vi "Main.vi"(11 "Module Admin":refnum<class "Delacor_lib_QMH_Module Admin.lvclass">) -> ()   [LabVIEW 2020, in "Manipulator.lvlib"]
doc: "This template is based off of the Queued Message Handler design pattern and the Queued Message Handler project template that ships with LabVIEW.\n\nThe main difference is that the queue is private to this module and communication between modules is performed via Broadcast and Request events.\n\nRequest events are wrapped in public API methods and are handled in the Event Handling Loop (EHL) of this VI. Any module can register for Broadcast events sent by this module. The EHL generates messages based on user interface actions.\n\nThe Message Handling Loop (MHL) processes messages generated by the EHL, or by other messages. The messages are string values, so new messages can be added easily to the Message Cases case structure in the MHL. Each message cluster can also provide an optional value for Message Data, which is a variant that can be converted to whatever message-specific data is required.\n_____\nBased on DQMH Project Template 6.0.0.91."
uses:
  Manipulator.lvlib
  <vilib>/Delacor/Delacor QMH/Libraries/Module Admin_class/Delacor_lib_QMH_Module Admin.lvclass
  Module Data--cluster.ctl
  <vilib>/Delacor/Delacor QMH/Libraries/Message Queue_class/Delacor_lib_QMH_Message Queue.lvclass/Delacor_lib_QMH_Message Queue.ctl
  Stop Argument--cluster.ctl
  <vilib>/Delacor/Delacor QMH/Libraries/Module Admin_class/Delacor_lib_QMH_Module Admin.lvclass/Delacor_lib_QMH_Module Admin.ctl
  Get Num Axes Argument--cluster.ctl
  Get Num Axes (Reply Payload)--cluster.ctl
  Get Position and Speed Argument--cluster.ctl
  Get Position and Speed (Reply Payload)--cluster.ctl
  Move Axis Argument--cluster.ctl
  Move Axis (Reply Payload)--cluster.ctl
  Get Status Argument--cluster.ctl
  Get Status (Reply Payload)--cluster.ctl
  Manipulator-CLIDriver/Manipulator Status.ctl
  Move Axis with Speed Argument--cluster.ctl
  Move Axis with Speed (Reply Payload)--cluster.ctl
  <vilib>/Utility/miscctls.llb/LVPointTypeDef.ctl
  <vilib>/Delacor/Delacor QMH/Libraries/Message Queue_class/Delacor_lib_QMH_Enqueue Message (Single).vi
  <vilib>/Delacor/Delacor QMH/Libraries/Module Admin_class/Delacor_lib_QMH_Get External Launch.vi
  <vilib>/Utility/error.llb/Error Cluster From Error Code.vi
  <vilib>/ErrorRing/Error Ring.xnode
  <vilib>/Delacor/Delacor QMH/Libraries/Message Queue_class/Delacor_lib_QMH_Message Queue.lvclass
  Manipulator-CLIDriver/Manipulator CLI Driver.lvlib
panel:
  out "error out":errorcluster
  out "Status":string
  in  "Simulate MHL Error":bool
  in  "Simulate EHL Error":bool
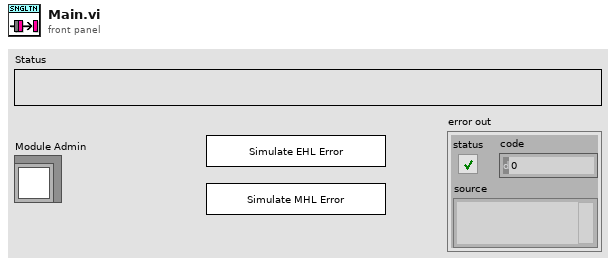
[diagram p1: front panel]
types:
  T1 = typedef "Manipulator.lvlib/Request Events--cluster.ctl" = cluster{"Stop Module":refnum<user-event>, "Show Panel":refnum<user-event>, "Hide Panel":refnum<user-event>, "Get Module Execution Status":refnum<user-event>, "Show Diagram":refnum<user-event>, "Get Num Axes":refnum<user-event>, "Get Position and Speed":refnum<user-event>, "Move Axis":refnum<user-event>, "Get Status":refnum<user-event>, "Move Axis with Speed":refnum<user-event>}
  T2 = typedef "Manipulator.lvlib/Module Data--cluster.ctl" = cluster{"Status":string}
  T3 = enum32{"invalid lock state", "Not Locked", "Locked (No Password)", "Password-protected"}
  T4 = typedef "Manipulator.lvlib/Stop Argument--cluster.ctl" = cluster{"Origin":string, "Exit via Stop Module Req?":bool, "Wait for Module to stop?":bool}
  T5 = typedef "Manipulator.lvlib/Get Num Axes Argument--cluster.ctl" = cluster{"Wait Notifier":refnum<notifier>, "wait for reply":bool}
  T6 = typedef "Manipulator.lvlib/Get Position and Speed Argument--cluster.ctl" = cluster{"Wait Notifier":refnum<notifier>, "wait for reply":bool}
  T7 = typedef "Manipulator.lvlib/Move Axis Argument--cluster.ctl" = cluster{"Axis":i32, "Position":dbl, "Wait Notifier":refnum<notifier>, "wait for reply":bool}
  T8 = typedef "Manipulator.lvlib/Get Status Argument--cluster.ctl" = cluster{"Wait Notifier":refnum<notifier>, "wait for reply":bool}
  T9 = typedef "Manipulator.lvlib/Move Axis with Speed Argument--cluster.ctl" = cluster{"Position":dbl, "Speed":dbl, "Axis":i32, "Wait Notifier":refnum<notifier>, "wait for reply":bool}
  T10 = typedef "LVPointTypeDef.ctl" = cluster{"Horizontal":i16, "Vertical":i16}
  T11 = enum32{"Invalid", "Standard", "Closed", "Hidden", "Minimized", "Maximized"}
  T12 = typedef "Manipulator.lvlib/Get Num Axes (Reply Payload)--cluster.ctl" = cluster{"Num Axes":i32, "Get Num Axes_error":errorcluster}
  T13 = typedef "Manipulator.lvlib/Get Position and Speed (Reply Payload)--cluster.ctl" = cluster{"Positions":dbl[], "Speeds":dbl[], "Get Position and Speed_error":errorcluster}
  T14 = typedef "Manipulator.lvlib/Move Axis (Reply Payload)--cluster.ctl" = cluster{"Move Axis_error":errorcluster}
  T15 = typedef "Manipulator.lvlib/Get Status (Reply Payload)--cluster.ctl" = cluster{"Status":T16, "Get Status_error":errorcluster}
  T16 = typedef "Manipulator CLI Driver.lvlib/Manipulator Status.ctl" = enum16{"Moving", "Done", "Aborted", "Error", "No Status"}
  T17 = typedef "Manipulator.lvlib/Move Axis with Speed (Reply Payload)--cluster.ctl" = cluster{"Move Axis with Speed_error":errorcluster}
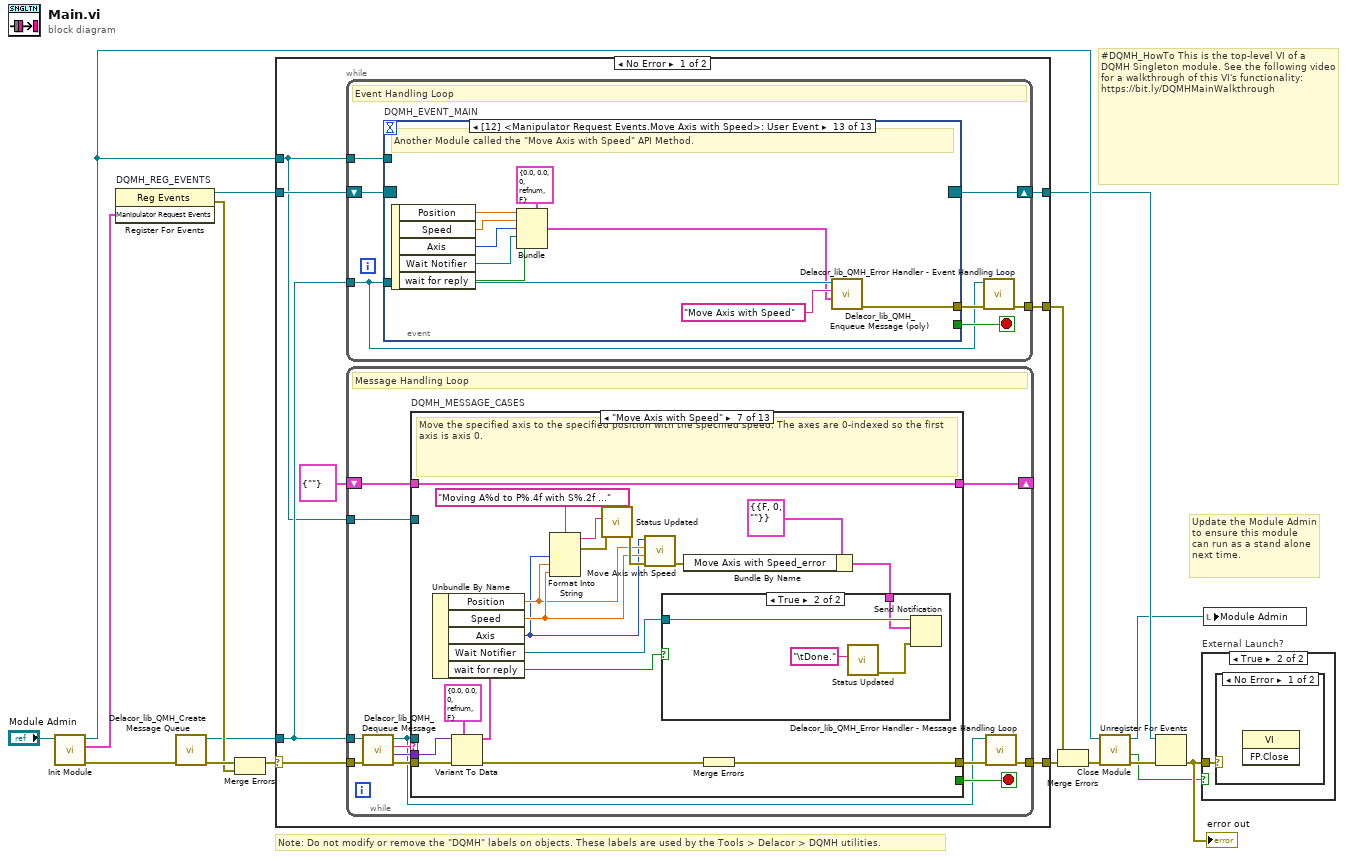
[diagram p0: block diagram]
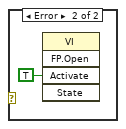
[diagram p3: hidden frame]
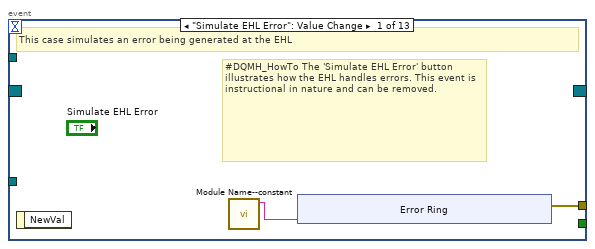
[diagram p4: hidden frame]
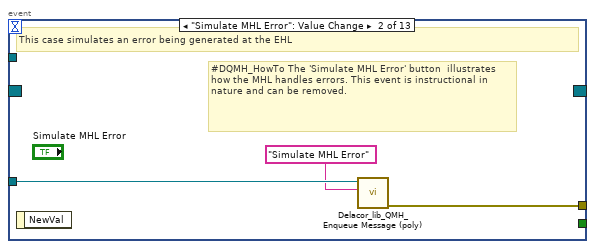
[diagram p5: hidden frame]
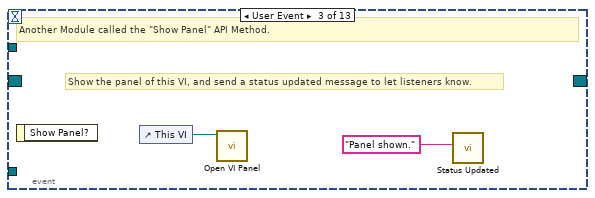
[diagram p6: hidden frame]
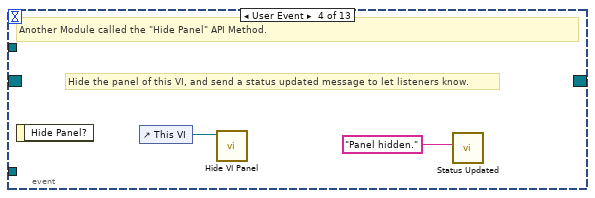
[diagram p7: hidden frame]
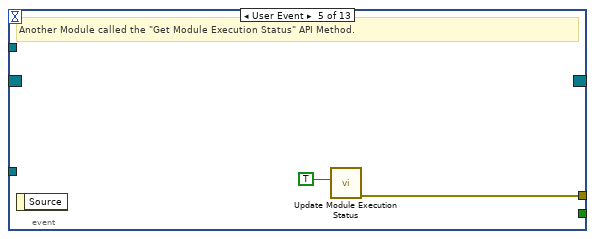
[diagram p8: hidden frame]
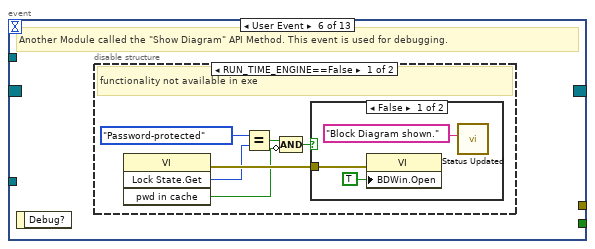
[diagram p9: hidden frame]
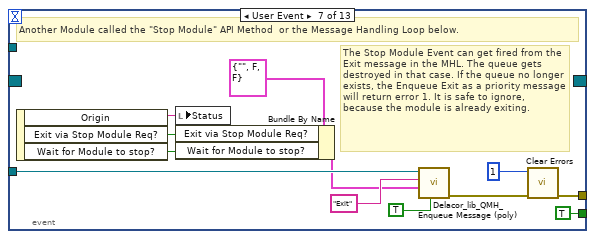
[diagram p12: hidden frame]
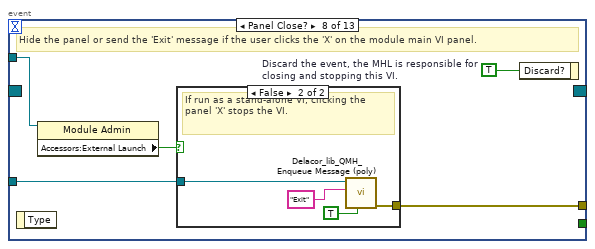
[diagram p13: hidden frame]
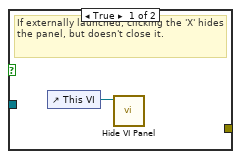
[diagram p14: hidden frame]
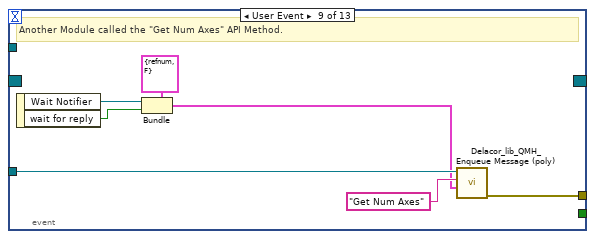
[diagram p15: hidden frame]
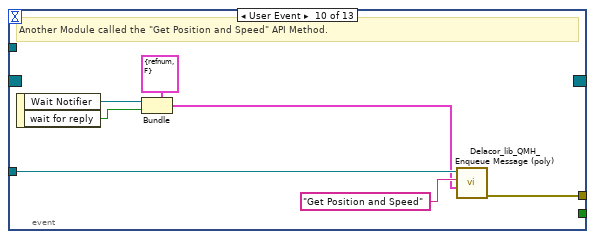
[diagram p16: hidden frame]
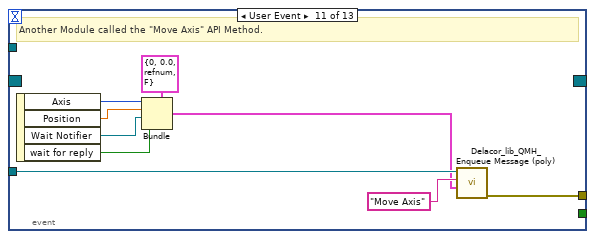
[diagram p17: hidden frame]
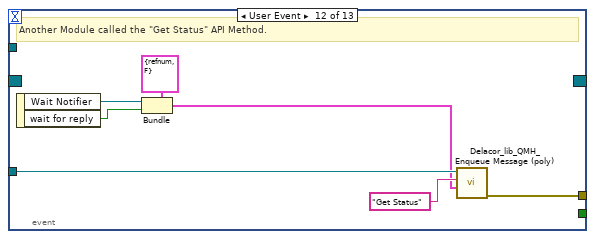
[diagram p18: hidden frame]
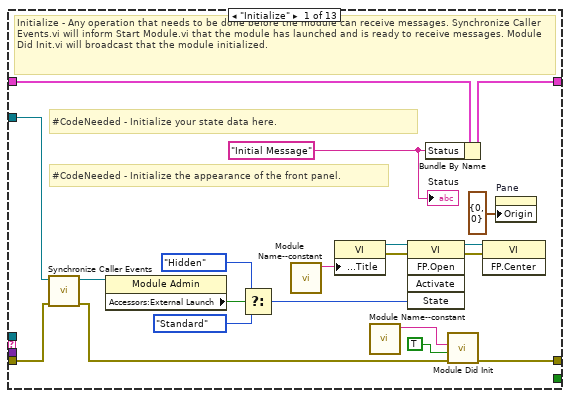
[diagram p19: hidden frame]
diagram:
  # "#DQMH_HowTo This is the top-level VI of a DQMH Singleton module. See the following video for a walkthrough of this VI's functionality: https://bit.ly/DQMHMainWalkthrough"
  # "Note: Do not modify or remove the \"DQMH\" labels on objects. These labels are used by the Tools > Delacor > DQMH utilities."
  # "Update the Module Admin to ensure this module can run as a stand alone next time."
  n1 = call "Init Module.vi"("Singleton Module Admin in"="Module Admin") -> ("error out"=w16:errorcluster, "Manipulator Request Events"=w5:T1, "Singleton Module Admin out"=w8:refnum<class "Delacor_lib_QMH_Module Admin.lvclass">)  [unwired: 8 in]
  n2 = register-events "DQMH_REG_EVENTS"(w5) -> (reference out=w6:refnum<event-registration>, error out=w9:errorcluster)  [unwired: 2 in]
  n3 = call <vilib>:"Delacor_lib_QMH_Create Message Queue.vi"("error in"=w16) -> ("error out"=w11:errorcluster, "Message Queue"=w4:refnum<class "Delacor_lib_QMH_Message Queue.lvclass">)  [unwired: 9 in]
  n4 = Merge Errors(w11, w9) -> (w10:errorcluster)
  n5 = case shown="No Error" w10 {
    selector: w10 -> [w23 w311]
    tunnel: [w25 w310] -> w17
    tunnel: [w22 w316] -> w7
    tunnel: w6 -> [w20 w316]
    tunnel: w4 -> [w19 w309]
    tunnel: [w24 _] -> w14
    tunnel: w8 -> [w18 w312]
    frame No Error {
      n6 = while {
        tunnel: w19 -> [w26]
        shift-right: [w29] -> w22
        shift-left: w20 -> [w30]
        tunnel: [w31] -> w24
        tunnel: w18 -> [w27]
        stop <- w28 stop-if-true
        # "Event Handling Loop"
        n7 = event "DQMH_EVENT_MAIN" shown="[12] <Manipulator Request Events.Move Axis with Speed>: User Event" {
          selector: w30 -> [_ _ _ _ _ _ _ _ _ _ _ _ _]
          dyn-events: [_ _ _ _ _ _ _ _ _ _ _ _ _] -> w29
          timeout: _ -> [_ _ _ _ _ _ _ _ _ _ _ _ _]
          tunnel: [_ _ _ _ _ _ TRUE ("Discard?") _ _ _ _ _ _] -> w28
          tunnel: w26 -> [_ w43 _ _ _ _ w67 w74 w88 w95 w104 w111 w121]
          tunnel: [w34 w44 _ _ w50 _ w70 w76 w82 w89 w96 w105 w112] -> w32
          tunnel: w27 -> [_ _ _ _ _ _ _ w73 _ _ _ _ _]
          event "Simulate EHL Error": Value Change {
            # "#DQMH_HowTo The 'Simulate EHL Error' button  illustrates how the EHL handles errors. This event is instructional in nature and can be removed."
            # "This case simulates an error being generated at the EHL"
            n8 = event-data() -> ()  [unwired: 1 in, 1 out]
            n9 = call "Module Name--constant.vi"() -> ("Module Name"=w33:string)  [unwired: 11 in]
            n10 = xnode "Error Ring"("parameter 0"=w33) -> ("error out"=w34:errorcluster)
          }
          event "Simulate MHL Error": Value Change {
            # "#DQMH_HowTo The 'Simulate MHL Error' button  illustrates how the MHL handles errors. This event is instructional in nature and can be removed."
            # "This case simulates an error being generated at the EHL"
            n11 = event-data() -> ()  [unwired: 1 in, 1 out]
            n12 = call-poly <vilib>:"Delacor_lib_QMH_Enqueue Message (poly).vi"("Message"="Simulate MHL Error", "Message Queue in"=w43) -> ("error out"=w44:errorcluster)  [unwired: 8 in, 1 out]
          }
          event User Event {
            # "Show the panel of this VI, and send a status updated message to let listeners know."
            # "Another Module called the \"Show Panel\" API Method."
            n13 = event-data() -> ()  [unwired: 1 in, 1 out]
            n14 = control-ref of="This VI"() -> (w46:refnum<vi>)
            n15 = call "Open VI Panel.vi"("VI"=w46) -> ()  [unwired: 10 in, 1 out]
            n16 = call "Status Updated.vi"("Status"="Panel shown." ("format string")) -> ()  [unwired: 10 in, 1 out]
          }
          event User Event {
            # "Hide the panel of this VI, and send a status updated message to let listeners know."
            # "Another Module called the \"Hide Panel\" API Method."
            n17 = event-data() -> ()  [unwired: 1 in, 1 out]
            n18 = control-ref of="This VI"() -> (w48:refnum<vi>)
            n19 = call "Hide VI Panel.vi"("VI"=w48) -> ()  [unwired: 10 in, 1 out]
            n20 = call "Status Updated.vi"("Status"="Panel hidden." ("format string")) -> ()  [unwired: 10 in, 1 out]
          }
          event User Event {
            # "Another Module called the \"Get Module Execution Status\" API Method."
            n21 = event-data() -> ()  [unwired: 1 in, 1 out]
            n22 = call "Update Module Execution Status.vi"("Running?"=TRUE) -> ("error out"=w50:errorcluster)  [unwired: 10 in]
          }
          event User Event {
            # "Another Module called the \"Show Diagram\" API Method. This event is used for debugging."
            n23 = event-data() -> ()  [unwired: 1 in, 1 out]
            n24 = disable-structure shown="RUN_TIME_ENGINE==False" {
              frame condition #0 (active) {
                # "functionality not available in exe"
                n25 = invoke class="VI" method="Lock State.Get"() -> (error out=w56:errorcluster, "Get Lock State"=w55:T3, "pwd in cache"=w52:bool)  [unwired: 4 in, 1 out]
                n26 = Equal?(x=T3."Password-protected", y=w55) -> (x = y?=w53:bool)
                n27 = Compound Arithmetic op=AND(w53, invert w52) -> (w51:bool)
                n28 = case shown="False" w51 {
                  tunnel: w56 -> [w59 _]
                  frame False {
                    n29 = property class="VI"(error in=w59, "BDWin.Open"=TRUE ("Block Diagram Window:Open")) -> ()  [unwired: 1 in, 2 out]
                    n30 = call "Status Updated.vi"("Status"="Block Diagram shown." ("format string")) -> ()  [unwired: 10 in, 1 out]
                  }
                  frame True {
                    # "Password-protected VI, and the password is not in the cache. Do not show the diagram."
                  }
                }
              }
              frame condition #1 {
              }
            }
          }
          event User Event {
            # "The Stop Module Event can get fired from the Exit message in the MHL. The queue gets destroyed in that case. If the queue no longer exists, the Enqueue Exit as a priority message will return error 1. It is safe to ignore, because the module is already exiting."
            # "Another Module called the \"Stop Module\" API Method  or the Message Handling Loop below."
            n31 = event-data() -> ("Origin"=w66:string, "Exit via Stop Module Req?"=w62:bool, "Wait for Module to stop?"=w61:bool)  [unwired: 1 in]
            n32 = local write "Status"(w66) -> ()
            n33 = Bundle By Name(cluster=T4 {"Origin"="", "Exit via Stop Module Req?"=FALSE, "Wait for Module to stop?"=FALSE} ("Stop Argument"), "Exit via Stop Module Req?"=w62, "Wait for Module to stop?"=w61) -> (w60:T4)
            n34 = call-poly <vilib>:"Delacor_lib_QMH_Enqueue Message (poly).vi"("Priority Message? (F)"=TRUE, "Message Data"=w60, "Message"="Exit", "Message Queue in"=w67) -> ("error out"=w71:errorcluster)  [unwired: 6 in, 1 out]
            n35 = call <vilib>:"Clear Errors.vi"("error in (no error)"=w71, "specific error code to clear (0: all)"=1) -> ("error out"=w70:errorcluster)  [unwired: 4 in, 1 out]
          }
          event Panel Close? {
            w75 = TRUE  # Discard the event, the MHL is responsible for closing and stopping this VI.
            # "Hide the panel or send the 'Exit' message if the user clicks the 'X' on the module main VI panel."
            n36 = event-data() -> ()  [unwired: 1 in, 1 out]
            n37 = property class="Module Admin"(reference=w73) -> ("Accessors:External Launch"=w72:bool)  [unwired: 1 in, 2 out]
            n38 = case shown="False" w72 {
              tunnel: w74 -> [_ w80]
              tunnel: [_ w81] -> w76
              frame True {
                # "If externally launched, clicking the 'X' hides the panel, but doesn't close it."
                n39 = control-ref of="This VI"() -> (w77:refnum<vi>)
                n40 = call "Hide VI Panel.vi"("VI"=w77) -> ()  [unwired: 10 in, 1 out]
              }
              frame False {
                # "If run as a stand-alone VI, clicking the panel 'X' stops the VI."
                n41 = call-poly <vilib>:"Delacor_lib_QMH_Enqueue Message (poly).vi"("Priority Message? (F)"=TRUE, "Message"="Exit", "Message Queue in"=w80) -> ("error out"=w81:errorcluster)  [unwired: 7 in, 1 out]
              }
            }
            n42 = event-data("Discard?"=w75) -> ()  [unwired: 1 in, 1 out]
          }
          event User Event {
            # "Another Module called the \"Get Num Axes\" API Method."
            n43 = event-data() -> ("Wait Notifier"=w84:refnum<notifier>, "wait for reply"=w83:bool)  [unwired: 1 in]
            n44 = Bundle(cluster=T5 {"Wait Notifier"=refnum, "wait for reply"=FALSE} ("Get Num Axes Argument"), "Wait Notifier"=w84, "wait for reply"=w83) -> (w85:T5)
            n45 = call-poly <vilib>:"Delacor_lib_QMH_Enqueue Message (poly).vi"("Message Data"=w85, "Message"="Get Num Axes", "Message Queue in"=w88) -> ("error out"=w82:errorcluster)  [unwired: 7 in, 1 out]
          }
          event User Event {
            # "Another Module called the \"Get Position and Speed\" API Method."
            n46 = event-data() -> ("Wait Notifier"=w91:refnum<notifier>, "wait for reply"=w90:bool)  [unwired: 1 in]
            n47 = Bundle(cluster=T6 {"Wait Notifier"=refnum, "wait for reply"=FALSE} ("Get Position and Speed Argument"), "Wait Notifier"=w91, "wait for reply"=w90) -> (w92:T6)
            n48 = call-poly <vilib>:"Delacor_lib_QMH_Enqueue Message (poly).vi"("Message Data"=w92, "Message"="Get Position and Speed", "Message Queue in"=w95) -> ("error out"=w89:errorcluster)  [unwired: 7 in, 1 out]
          }
          event User Event {
            # "Another Module called the \"Move Axis\" API Method."
            n49 = event-data() -> ("Axis"=w100:i32, "Position"=w99:dbl, "Wait Notifier"=w98:refnum<notifier>, "wait for reply"=w97:bool)  [unwired: 1 in]
            n50 = Bundle(cluster=T7 {"Axis"=0, "Position"=0.0, "Wait Notifier"=refnum, "wait for reply"=FALSE} ("Move Axis Argument"), "Axis"=w100, "Position"=w99, "Wait Notifier"=w98, "wait for reply"=w97) -> (w101:T7)
            n51 = call-poly <vilib>:"Delacor_lib_QMH_Enqueue Message (poly).vi"("Message Data"=w101, "Message"="Move Axis", "Message Queue in"=w104) -> ("error out"=w96:errorcluster)  [unwired: 7 in, 1 out]
          }
          event User Event {
            # "Another Module called the \"Get Status\" API Method."
            n52 = event-data() -> ("Wait Notifier"=w107:refnum<notifier>, "wait for reply"=w106:bool)  [unwired: 1 in]
            n53 = Bundle(cluster=T8 {"Wait Notifier"=refnum, "wait for reply"=FALSE} ("Get Status Argument"), "Wait Notifier"=w107, "wait for reply"=w106) -> (w108:T8)
            n54 = call-poly <vilib>:"Delacor_lib_QMH_Enqueue Message (poly).vi"("Message Data"=w108, "Message"="Get Status", "Message Queue in"=w111) -> ("error out"=w105:errorcluster)  [unwired: 7 in, 1 out]
          }
          event User Event {
            # "Another Module called the \"Move Axis with Speed\" API Method."
            n55 = event-data() -> ("Position"=w117:dbl, "Speed"=w116:dbl, "Axis"=w115:i32, "Wait Notifier"=w114:refnum<notifier>, "wait for reply"=w113:bool)  [unwired: 1 in]
            n56 = Bundle(cluster=T9 {"Position"=0.0, "Speed"=0.0, "Axis"=0, "Wait Notifier"=refnum, "wait for reply"=FALSE} ("Move Axis with Speed Argument"), "Position"=w117, "Speed"=w116, "Axis"=w115, "Wait Notifier"=w114, "wait for reply"=w113) -> (w118:T9)
            n57 = call-poly <vilib>:"Delacor_lib_QMH_Enqueue Message (poly).vi"("Message Data"=w118, "Message"="Move Axis with Speed", "Message Queue in"=w121) -> ("error out"=w112:errorcluster)  [unwired: 7 in, 1 out]
          }
        }
        n58 = call-dynamic "Delacor_lib_QMH_Error Handler - Event Handling Loop.vi"("error in"=w32, "Message Queue in"=w26) -> ("dup error in"=w31:errorcluster)  [unwired: 8 in, 1 out]
      }
      n59 = while {
        tunnel: w19 -> [w124]
        shift-right: [w128] -> _
        shift-left: T2 {"Status"=""} ("Data Cluster") -> [w129]
        tunnel: w23 -> [w132]
        tunnel: [w130] -> w25
        tunnel: w18 -> [w122]
        stop <- w127 stop-if-true
        # "Message Handling Loop"
        n60 = call-dynamic "Delacor_lib_QMH_Dequeue Message.vi"("error in"=w132, "Message Queue in"=w124) -> ("error out"=w131:errorcluster, "Message Data"=w125:variant, "Message"=w126:string, "Message Queue out"=w123:refnum<class "Delacor_lib_QMH_Message Queue.lvclass">)  [unwired: 6 in]
        n61 = case "DQMH_MESSAGE_CASES" shown="\"Move Axis with Speed\"" w126 {
          selector: w126 -> [_ _ _ _ _ _ _ _ _ _ _ _ w296]
          tunnel: w123 -> [_ _ _ _ _ _ _ _ _ _ w266 w288 _]
          tunnel: w131 -> [w151 w155 w168 w184 w204 w221 w242 w249 w251 w256 w273 w294 w298]
          tunnel: [w149 w155 w158 w174 w194 w211 w232 w248 w251 w255 w269 w291 w299] -> w133
          tunnel: w129 -> [w140 w154 w167 w183 w203 w220 w241 w247 w250 w253 w268 w287 w297]
          tunnel: [w139 w154 w167 w183 w203 w220 w241 w247 w250 w253 w268 w287 w297] -> w128
          tunnel: [_ _ _ _ _ _ _ _ _ _ _ w286 _] -> w127
          tunnel: w125 -> [_ _ w165 w181 w201 w218 w239 _ _ _ w267 w285 _]
          tunnel: w122 -> [w141 _ _ _ _ _ _ _ _ _ w265 w280 _]
          frame "Initialize" {
            w135 = "Initial Message" ("Initial Message")
            # "#CodeNeeded - Initialize the appearance of the front panel."
            # "#CodeNeeded - Initialize your state data here."
            # "Initialize - Any operation that needs to be done before the module can receive messages. Synchronize Caller Events.vi will inform Start Module.vi that the module has launched and is ready to receive messages. Module Did Init.vi will broadcast that the module initialized."
            n62 = call "Synchronize Caller Events.vi"("error in (no error)"=w151, "Singleton Module Admin in"=w141) -> ("error out"=w150:errorcluster, "Singleton Module Admin out"=w136:refnum<class "Delacor_lib_QMH_Module Admin.lvclass">)  [unwired: 8 in]
            n63 = property class="Module Admin"(reference=w136) -> ("Accessors:External Launch"=w145:bool)  [unwired: 1 in, 2 out]
            n64 = Select(t=T11."Hidden" ("State"), s=w145, f=T11."Standard" ("State")) -> (s? t:f=w142:T11)
            n65 = call "Module Name--constant.vi"() -> ("Module Name"=w148:string)  [unwired: 11 in]
            n66 = property class="VI"("Front Panel.Title"=w148) -> (reference out=w147:refnum<vi>, error out=w153:errorcluster)  [unwired: 2 in]
            n67 = call "Module Name--constant.vi"() -> ("Module Name"=w137:string)  [unwired: 11 in]
            n68 = invoke class="VI" method="FP.Open"(reference=w147, error in=w153, "State"=w142) -> (reference out=w146:refnum<vi>, error out=w152:errorcluster)  [unwired: 2 in, 3 out]
            n69 = Bundle By Name(cluster=w140, "Status"=w135) -> (w139:T2)
            n70 = call "Module Did Init.vi"("error in (no error)"=w150, "Initialized?"=TRUE, "Origin"=w137) -> ("error out"=w149:errorcluster)  [unwired: 8 in]
            n71 = invoke class="VI" method="FP.Center"(reference=w146, error in=w152) -> ()  [unwired: 1 in, 3 out]
            n72 = property on="Pane" class="Pane"("Origin"=T10 {"Horizontal"=0, "Vertical"=0}) -> ()  [unwired: 2 in, 2 out]
            "Status" <- w135
          }
          frame "---Module Specific---" {
            # "Separator -- The following cases handle messages specific to this Module."
          }
          frame "Get Num Axes" {
            # "Get the number of axes of the manipulator."
            n73 = Variant To Data(error in=w168, type=T5 {"Wait Notifier"=refnum, "wait for reply"=FALSE} ("Get Num Axes Argument"), Variant=w165) -> (data=w163:T5, error out=w166:errorcluster)
            n74 = call "Get Num Axes.vi"() -> ("error out"=w157:errorcluster, "num-axes"=w156:i32)  [unwired: 10 in]
            n75 = Unbundle By Name(w163) -> ("Wait Notifier"=w162:refnum<notifier>, "wait for reply"=w161:bool)
            n76 = Merge Errors(w166) -> (w158:errorcluster)
            n77 = Bundle By Name(cluster=T12 {"Num Axes"=0, "Get Num Axes_error"={"status"=FALSE, "code"=0, "source"=""}} ("Get Num Axes (Reply Payload)"), "Num Axes"=w156, "Get Num Axes_error"=w157) -> (w160:T12)
            n78 = case shown="True" w161 {
              tunnel: w162 -> [_ w170]
              tunnel: w160 -> [_ w169]
              frame False {
              }
              frame True {
                n79 = Send Notification(notification=w169, notifier=w170) -> ()  [unwired: 1 in, 2 out]
              }
            }
            n80 = call "Broadcast Num Axes.vi"("Reply Payload"=w160) -> ()  [unwired: 10 in, 1 out]
          }
          frame "Get Position and Speed" {
            # "Get the position and speed of all axes as two separate arrays."
            n81 = Variant To Data(error in=w184, type=T6 {"Wait Notifier"=refnum, "wait for reply"=FALSE} ("Get Position and Speed Argument"), Variant=w181) -> (data=w179:T6, error out=w182:errorcluster)
            n82 = call "Get Position.vi"() -> ("error out"=w171:errorcluster, "speeds"=w172:dbl[], "positions"=w173:dbl[])  [unwired: 9 in]
            n83 = Unbundle By Name(w179) -> ("Wait Notifier"=w178:refnum<notifier>, "wait for reply"=w177:bool)
            n84 = Bundle By Name(cluster=T13 {"Positions"=[], "Speeds"=[], "Get Position and Speed_error"={"status"=FALSE, "code"=0, "source"=""}} ("Get Position and Speed (Reply Payload)"), "Positions"=w173, "Speeds"=w172, "Get Position and Speed_error"=w171) -> (w176:T13)
            n85 = case shown="True" w177 {
              tunnel: w178 -> [_ w186]
              tunnel: w176 -> [_ w185]
              frame False {
              }
              frame True {
                n86 = Send Notification(notification=w185, notifier=w186) -> ()  [unwired: 1 in, 2 out]
              }
            }
            n87 = Merge Errors(w182) -> (w174:errorcluster)
            n88 = call "Broadcast Position and Speed.vi"("Reply Payload"=w176) -> ()  [unwired: 10 in, 1 out]
          }
          frame "Move Axis" {
            # "Move the specified axis to the specified position. The axes are 0-indexed, so the first axis is 0."
            n89 = Variant To Data(error in=w204, type=T7 {"Axis"=0, "Position"=0.0, "Wait Notifier"=refnum, "wait for reply"=FALSE} ("Move Axis Argument"), Variant=w201) -> (data=w199:T7, error out=w202:errorcluster)
            n90 = Unbundle By Name(w199) -> ("Axis"=w187:i32, "Position"=w188:dbl, "Wait Notifier"=w198:refnum<notifier>, "wait for reply"=w197:bool)
            n91 = Format Into String(format string="Moving A%d to P%.4f ...", w187, w188) -> (resulting string=w190:string, error out=w191:errorcluster)  [unwired: 2 in]
            n92 = call "Status Updated.vi"("error in (no error)"=w191, "Status"=w190) -> ("error out"=w192:errorcluster)  [unwired: 9 in]
            n93 = call "Move Axis.vi"("error in (no error)"=w192, "Position"=w188, "Axis"=w187) -> ("error out"=w193:errorcluster)  [unwired: 8 in]
            n94 = Merge Errors(w202) -> (w194:errorcluster)
            n95 = Bundle By Name(cluster=T14 {"Move Axis_error"={"status"=FALSE, "code"=0, "source"=""}} ("Move Axis (Reply Payload)"), "Move Axis_error"=w193) -> (w196:T14)
            n96 = case shown="True" w197 {
              tunnel: w198 -> [_ w208]
              tunnel: w196 -> [_ w207]
              frame False {
              }
              frame True {
                n97 = call "Status Updated.vi"("Status"="\tDone.") -> ("error out"=w206:errorcluster)  [unwired: 10 in]
                n98 = Send Notification(notification=w207, notifier=w208, error in (no error)=w206) -> ()  [unwired: 2 out]
              }
            }
          }
          frame "Get Status" {
            # "Get the Status of the Manipulator."
            n99 = Variant To Data(error in=w221, type=T8 {"Wait Notifier"=refnum, "wait for reply"=FALSE} ("Get Status Argument"), Variant=w218) -> (data=w216:T8, error out=w219:errorcluster)
            n100 = Unbundle By Name(w216) -> ("Wait Notifier"=w215:refnum<notifier>, "wait for reply"=w214:bool)
            n101 = call "Get Status.vi"() -> ("error out"=w209:errorcluster, "Status"=w210:T16)  [unwired: 10 in]
            n102 = Merge Errors(w219) -> (w211:errorcluster)
            n103 = Bundle By Name(cluster=T15 {"Status"=enum."Moving", "Get Status_error"={"status"=FALSE, "code"=0, "source"=""}} ("Get Status (Reply Payload)"), "Status"=w210, "Get Status_error"=w209) -> (w213:T15)
            n104 = case shown="True" w214 {
              tunnel: w215 -> [_ w223]
              tunnel: w213 -> [_ w222]
              frame False {
              }
              frame True {
                n105 = Send Notification(notification=w222, notifier=w223) -> ()  [unwired: 1 in, 2 out]
              }
            }
            n106 = call "Broadcast Status.vi"("Reply Payload"=w213) -> ()  [unwired: 10 in, 1 out]
          }
          frame "Move Axis with Speed" {
            # "Move the specified axis to the specified position with the specified speed. The axes are 0-indexed so the first axis is axis 0."
            n107 = Variant To Data(error in=w242, type=T9 {"Position"=0.0, "Speed"=0.0, "Axis"=0, "Wait Notifier"=refnum, "wait for reply"=FALSE} ("Move Axis with Speed Argument"), Variant=w239) -> (data=w237:T9, error out=w240:errorcluster)
            n108 = Unbundle By Name(w237) -> ("Position"=w225:dbl, "Speed"=w226:dbl, "Axis"=w224:i32, "Wait Notifier"=w236:refnum<notifier>, "wait for reply"=w235:bool)
            n109 = Format Into String(format string="Moving A%d to P%.4f with S%.2f ...", w224, w225, w226) -> (resulting string=w228:string, error out=w227:errorcluster)  [unwired: 2 in]
            n110 = call "Status Updated.vi"("error in (no error)"=w227, "Status"=w228) -> ("error out"=w229:errorcluster)  [unwired: 9 in]
            n111 = call "Move Axis with Speed.vi"("error in (no error)"=w229, "Speed"=w226, "Position"=w225, "Axis"=w224) -> ("error out"=w231:errorcluster)  [unwired: 7 in]
            n112 = Bundle By Name(cluster=T17 {"Move Axis with Speed_error"={"status"=FALSE, "code"=0, "source"=""}} ("Move Axis with Speed (Reply Payload)"), "Move Axis with Speed_error"=w231) -> (w234:T17)
            n113 = case shown="True" w235 {
              tunnel: w236 -> [_ w246]
              tunnel: w234 -> [_ w245]
              frame False {
              }
              frame True {
                n114 = call "Status Updated.vi"("Status"="\tDone.") -> ("error out"=w244:errorcluster)  [unwired: 10 in]
                n115 = Send Notification(notification=w245, notifier=w246, error in (no error)=w244) -> ()  [unwired: 2 out]
              }
            }
            n116 = Merge Errors(w240) -> (w232:errorcluster)
          }
          frame "---Copy This Frame---" {
            # "Duplicate this frame when creating new messages.  Change this comment in the duplicated frame to describe this message."
            n117 = Merge Errors(w249) -> (w248:errorcluster)
          }
          frame "---Exit and Error Handling---" {
            # "Separator - The following cases handle errors and exit messages."
          }
          frame "Simulate MHL Error" {
            # "#DQMH_HowTo The 'Simulate MHL Error' button  illustrates how the MHL handles errors. This event is instructional in nature and can be removed."
            # "Simulate an error occurring at the MHL"
            n118 = call "Module Name--constant.vi"() -> ("Module Name"=w252:string)  [unwired: 11 in]
            n119 = xnode "Error Ring"("parameter 0"=w252) -> ("error out"=w254:errorcluster)
            n120 = Merge Errors(w256, w254) -> (w255:errorcluster)
          }
          frame "Error" {
            # "#CodeRecommended - If you ever change the name of this \"Error\" message, you'll need to update the name in the Check Loop Error.vi as well."
            # "#CodeRecommended - If the module is running in standalone mode (External Launch = FALSE), this code will pop up an error dialog and call the 'Exit' message if an error occurs. Add more fine-grained error handling here."
            # "Error - Check the error message data and respond accordingly. This message is sent by the \"Error Handler\" VIs at the end of each loop in this application."
            n121 = property class="Module Admin"(reference=w265) -> ("Accessors:External Launch"=w264:bool)  [unwired: 1 in, 2 out]
            n122 = Variant To Data(error in=w273, type=errorcluster {"status"=FALSE, "code"=0, "source"=""} ("error constant"), Variant=w267) -> (data=w274:errorcluster, error out=w271:errorcluster)
            n123 = call "Error Reported.vi"("Error"=w274) -> ()  [unwired: 10 in, 1 out]
            n124 = case shown="False" w264 {
              tunnel: [w279 _] -> w270
              tunnel: w266 -> [w277 _]
              tunnel: w274 -> [w278 _]
              frame False {
                # "If the module is running standalone, then pop up an error dialog and call the \"Exit\" message."
                n125 = call <vilib>:"Simple Error Handler.vi"("error in (no error)"=w278) -> ()  [unwired: 4 in, 5 out]
                n126 = call-poly <vilib>:"Delacor_lib_QMH_Enqueue Message (poly).vi"("Priority Message? (F)"=TRUE, "Message"="Exit", "Message Queue in"=w277) -> ("error out"=w279:errorcluster)  [unwired: 7 in, 1 out]
              }
              frame True {
                # "If the module was launched externally, calling the Error Reported broadcast VI is the only action performed by the \"Error\" message. The module's caller can then process the error appropriately."
              }
            }
            n127 = Merge Errors(w271, w270) -> (w269:errorcluster)
            n128 = local write "error out"(w269) -> ()
          }
          frame "Exit" {
            w284 = 91  # 91: not all Exit messages will have an argument
            w286 = TRUE  # Stop the VI
            # "Release the message queue reference"
            # "#CodeNeeded - Add any required cleanup code here"
            # "Exit - Exit the application."
            n129 = Variant To Data(error in=w294, type=T4 {"Origin"="", "Exit via Stop Module Req?"=FALSE, "Wait for Module to stop?"=FALSE} ("Stop Argument"), Variant=w285) -> (data=w282:T4, error out=w290:errorcluster)
            n130 = call <vilib>:"Clear Errors.vi"("error in (no error)"=w290, "specific error code to clear (0: all)"=w284) -> ("error out"=w293:errorcluster)  [unwired: 4 in, 1 out]
            n131 = control-ref of="This VI"() -> (w281:refnum<vi>)
            n132 = call-dynamic "Delacor_lib_QMH_Release Message Queue.vi"("error in"=w293, "Message Queue"=w288) -> ("error out"=w292:errorcluster)  [unwired: 9 in]
            n133 = call "Handle Exit.vi"("Stop Argument"=w282, "Admin in"=w280, "VI reference"=w281) -> ("error out"=w289:errorcluster)  [unwired: 7 in, 1 out]
            n134 = Merge Errors(w292, w289) -> (w291:errorcluster)
          }
          frame Default {
            # "'Default' case only runs if there is a message that isn't defined in any of the other cases.  Output a programming error."
            n135 = call "Module Name--constant.vi"() -> ("Module Name"=w295:string)  [unwired: 11 in]
            n136 = xnode "Error Ring"("parameter 0"=w296, "parameter 1"=w295) -> ("error out"=w300:errorcluster)
            n137 = Merge Errors(w298, w300) -> (w299:errorcluster)
          }
        }
        n138 = call-dynamic "Delacor_lib_QMH_Error Handler - Message Handling Loop.vi"("error in"=w133, "Message Queue in"=w123) -> ("dup error in"=w130:errorcluster)  [unwired: 8 in, 1 out]
      }
    }
    frame Error {
      # "Synchronize Caller Events.vi will inform Start Module.vi that the module has launched and will let the code calling Start Module.vi register for broadcasts and would permit the caller receive the broadcast that an error occurred at launch time."
      n139 = call-dynamic "Delacor_lib_QMH_Release Message Queue.vi"("error in"=w311, "Message Queue"=w309) -> ("error out"=w310:errorcluster)  [unwired: 9 in]
      n140 = call "Synchronize Caller Events.vi"("Singleton Module Admin in"=w312) -> ("error out"=w317:errorcluster)  [unwired: 9 in, 1 out]
      n141 = call "Module Name--constant.vi"() -> ("Module Name"=w315:string)  [unwired: 11 in]
      n142 = Format Into String(format string="An error occurred during initialization. %s is no longer running.", w315) -> (resulting string=w313:string)  [unwired: 2 in, 1 out]
      n143 = Merge Errors(w310, w317) -> (w318:errorcluster)
      n144 = call "Error Reported.vi"("Additional Information"=w313, "Error"=w318) -> ()  [unwired: 9 in, 1 out]
    }
  }
  n145 = Merge Errors(w14, w17) -> (w13:errorcluster)
  n146 = call "Close Module.vi"("error in (no error)"=w13, "Module Admin in"=w8) -> ("error out"=w15:errorcluster, "External Launch"=w1:bool, "Module Admin out"=w2:refnum<class "Delacor_lib_QMH_Module Admin.lvclass">)  [unwired: 7 in]
  n147 = Unregister For Events(event registration refnum=w7, error in=w15) -> (error out=w12:errorcluster)
  "error out" <- w12
  n148 = case "External Launch?" shown="True" w1 {
    tunnel: w12 -> [_ w319]
    frame False {
    }
    frame True {
      n149 = case shown="No Error" w319 {
        frame No Error {
          n150 = invoke class="VI" method="FP.Close"() -> ()  [unwired: 3 in, 3 out]
        }
        frame Error {
          n151 = invoke class="VI" method="FP.Open"("Activate"=TRUE ("Activate?")) -> ()  [unwired: 4 in, 5 out]
        }
      }
    }
  }
  n152 = local write "Module Admin"(w2) -> ()
